vi "GLOBAL_timing_data.vi"(4 "Data in":u16[](array[numeric]), 5 "State":enum16{"Initialise", "Write", "Read"}(ring)) -> (1 "Valid Read?":bool, 2 "Data out":u16[](array[numeric]))   [LabVIEW 2014]
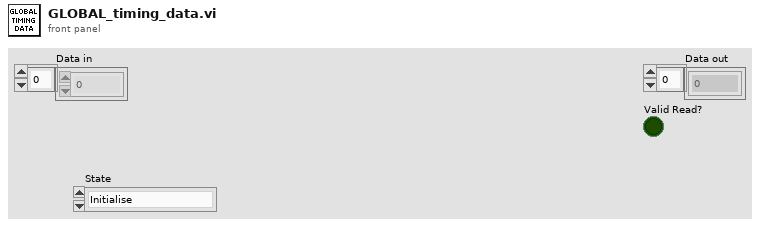
[diagram p1: front panel]
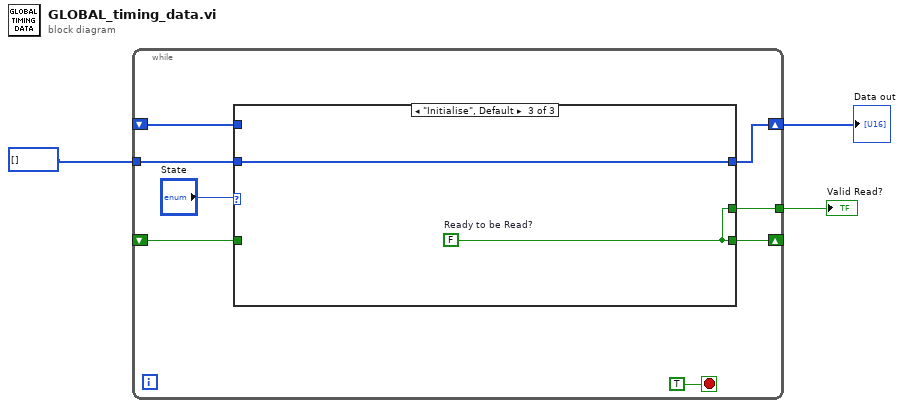
[diagram p0: block diagram]
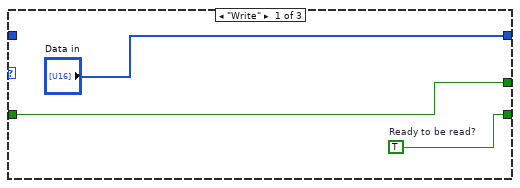
[diagram p2: hidden frame]
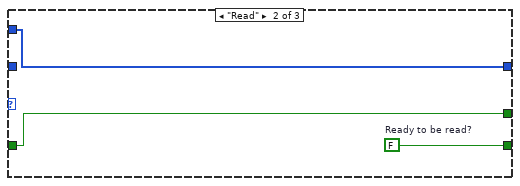
[diagram p3: hidden frame]
diagram:
  n1 = while {
    shift-right: [w8] -> w3
    shift-left: _ -> [w7]
    tunnel: u16[] [] ("Data in") -> [w9]
    shift-right: [w4] -> _
    shift-left: _ -> [w5]
    tunnel: [w6] -> w1
    stop <- TRUE stop-if-true
    n2 = case shown="\"Initialise\", Default" "State" {
      tunnel: w9 -> [_ _ w19]
      tunnel: ["Data in" w17 w19] -> w8
      tunnel: w7 -> [_ w17 _]
      tunnel: [w13 w16 w18] -> w6
      tunnel: w5 -> [w13 w16 _]
      tunnel: [w12 w15 w18] -> w4
      frame "Write" {
        w12 = TRUE  # Ready to be read?
      }
      frame "Read" {
        w15 = FALSE  # Ready to be read?
      }
      frame "Initialise", Default {
        w18 = FALSE  # Ready to be Read?
      }
    }
  }
  "Data out" <- w3
  "Valid Read?" <- w1
